vi "week04_Ex04.vi"() -> ()   [LabVIEW 2017]
uses:
  <vilib>/regexp/Match Regular Expression.xnode
panel:
  in  "stop":bool
  out "S Char":bool
  out "Number":bool
  out "low":bool
  out "Upper":bool
  out "length":dbl
  out "Length":bool
  in  "String":string
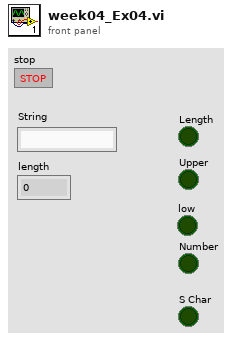
[diagram p1: front panel]
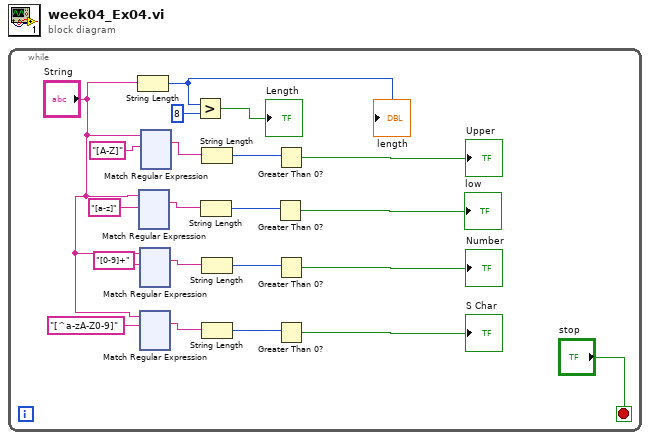
[diagram p0: block diagram]
diagram:
  n1 = while {
    stop <- "stop" stop-if-true
    n2 = String Length(string="String") -> (length=w16:i32)
    "length" <- w16
    n3 = xnode "Match Regular Expression"("input string"="String", "regular expression"="[a-z]") -> ("whole match"=w4:string)  [unwired: 4 in, 4 out]
    n4 = xnode "Match Regular Expression"("input string"="String", "regular expression"="[0-9]+") -> ("whole match"=w3:string)  [unwired: 4 in, 4 out]
    n5 = xnode "Match Regular Expression"("input string"="String", "regular expression"="[^a-zA-Z0-9]") -> ("whole match"=w2:string)  [unwired: 4 in, 4 out]
    n6 = xnode "Match Regular Expression"("input string"="String", "regular expression"="[A-Z]") -> ("whole match"=w13:string)  [unwired: 4 in, 4 out]
    n7 = Greater?(x=w16, y=8) -> (0:→"Length":bool)
    n8 = String Length(string=w4) -> (length=w9:i32)
    n9 = String Length(string=w13) -> (length=w12:i32)
    n10 = String Length(string=w3) -> (length=w8:i32)
    n11 = String Length(string=w2) -> (length=w5:i32)
    n12 = Greater Than 0?(x=w9) -> (x > 0?=→"low":bool)
    n13 = Greater Than 0?(x=w12) -> (x > 0?=→"Upper":bool)
    n14 = Greater Than 0?(x=w8) -> (x > 0?=→"Number":bool)
    n15 = Greater Than 0?(x=w5) -> (x > 0?=→"S Char":bool)
  }
